vi "Sorted Particle Report.vi"(3 "Min Area Size %":dbl, 4 "Particle Count Limit":i32=2147483647, 5 "Pixel Measurements":T2[](array[typedef])=[35, 4, 5, 6, 7] items=["Center of Mass X", "Center of Mass Y", "First Pixel X", "First Pixel Y", "Bounding Rect Left", "Bounding Rect Top", "Bounding Rect Right", "Bounding Rect Bottom", "Max Feret Diameter Start X", "Max Feret Diameter Start Y", "Max Feret Diameter End X", "Max Feret Diameter End Y", "Max Horiz. Segment Length Left", "Max Horiz. Segment Length Right", "Max Horiz. Segment Length Row", "-", "Bounding Rect Width", "Bounding Rect Height", "Bounding Rect Diagonal", "Perimeter", "Convex Hull Perimeter", "Holes' Perimeter", "Max Feret Diameter", "Equivalent Ellipse Major Axis", "Equivalent Ellipse Minor Axis", "Equivalent Ellipse Minor Axis (Feret)", "Equivalent Rect Long Side", "Equivalent Rect Short Side", "Equivalent Rect Diagonal", "Equivalent Rect Short Side (Feret)", "Average Horiz. Segment Length", "Average Vert. Segment Length", "Hydraulic Radius", "Waddel Disk Diameter", "-", "Area", "Holes' Area", "Particle & Holes' Area", "Convex Hull Area", "Image Area", "-", "Number of Holes", "Number of Horiz. Segments", "Number of Vert. Segments", "-", "Orientation", "Max Feret Diameter Orientation", "-", "% Area/Image Area", "% Area/(Particle & Holes' Area)", "Ratio of Equivalent Ellipse Axes", "Ratio of Equivalent Rect Sides", "-", "Elongation Factor", "Compactness Factor", "Heywood Circularity Factor", "Type Factor", "-", "Sum X", "Sum Y", "Sum XX", "Sum XY", "Sum YY", "Sum XXX", "Sum XXY", "Sum XYY", "Sum YYY", "-", "Moment of Inertia XX", "Moment of Inertia XY", "Moment of Inertia YY", "Moment of Inertia XXX", "Moment of Inertia XXY", "Moment of Inertia XYY", "Moment of Inertia YYY", "Norm. Moment of Inertia XX", "Norm. Moment of Inertia XY", "Norm. Moment of Inertia YY", "Norm. Moment of Inertia XXX", "Norm. Moment of Inertia XXY", "Norm. Moment of Inertia XYY", "Norm. Moment of Inertia YYY", "Hu Moment 1", "Hu Moment 2", "Hu Moment 3", "Hu Moment 4", "Hu Moment 5", "Hu Moment 6", "Hu Moment 7"], 6 "Image in":T3) -> (0 "limits":T1, 1 "Sorted Data":dbl[][](array[numeric]), 2 "Particles":i32)   [LabVIEW 2019]
doc: "Returns the requested measurements of a binary image sorted by the first parameter (often size), and limiting the rows in the 2D array by count and by size. Pass infinity to count to avoid a limit. Pass zero to size to avoid a limit."
uses:
  <vilib>/vision/Image Controls.llb/IMAQ Image.ctl
  <vilib>/vision/NI_Vision_Development_Module.lvlib
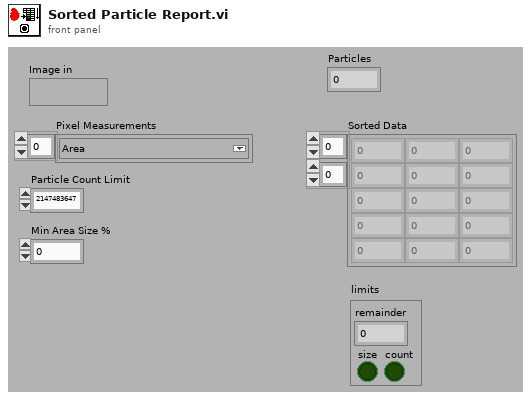
[diagram p1: front panel]
types:
  T1 = cluster{"remainder":i32, "size":bool, "count":bool}
  T2 = typedef "Particle Parameters" = i32
  T3 = typedef "IMAQ Image.ctl" = refnum<image>
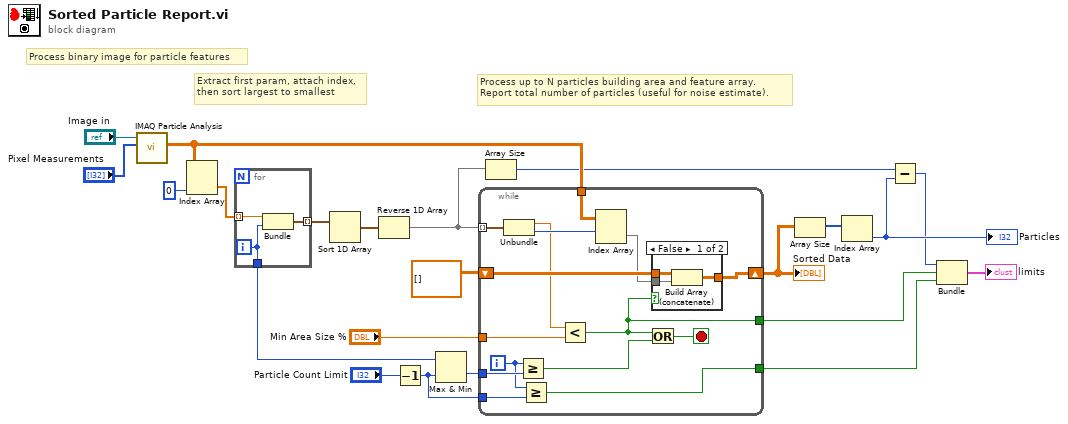
[diagram p0: block diagram]
diagram:
  # "Process up to N particles building area and feature array.\nReport total number of particles (useful for noise estimate)."
  # "Process binary image for particle features"
  # "Extract first param, attach index,\nthen sort largest to smallest"
  n1 = call "IMAQ Particle Analysis"("Pixel Measurements"="Pixel Measurements", "Image"="Image in") -> ("Particle Measurements (Pixels)"=w16:dbl[][])  [unwired: 3 in, 6 out]
  n2 = Index Array(array=w16, index (col)=0 ("disabled index (col)")) -> (element=w19:dbl[])  [unwired: 1 in]
  n3 = for {
    tunnel: w19 -> [w25] mode=indexing
    tunnel: [w24] -> w20 mode=indexing
    tunnel: [w23] -> w9
    i -> [w23]
    n4 = Bundle("Numeric"=w25, w23) -> (w24:cluster{"Numeric":dbl, i32})  [unwired: 1 out]
  }
  n5 = Sort 1D Array(array=w20) -> (sorted array=w21:cluster{"Numeric":dbl, i32}[])
  n6 = Reverse 1D Array(array=w21) -> (reversed array=w8:cluster{"Numeric":dbl, i32}[])
  n7 = Decrement(x="Particle Count Limit") -> (x-1=w1:i32)
  n8 = Max & Min(x=w9, y=w1) -> (min(x,y)=w10:i32)  [unwired: 1 out]
  n9 = while {
    tunnel: w16 -> [w39]
    tunnel: w8 -> [w38] mode=indexing
    shift-right: [w35] -> w12
    shift-left: dbl[][] [] -> [w37]
    tunnel: w10 -> [w34]
    tunnel: "Min Area Size %" -> [w32]
    tunnel: [w26] -> w3
    tunnel: [w29] -> w4
    tunnel: w1 -> [w28]
    i -> [w27]
    stop <- w31 stop-if-true
    n10 = Unbundle(w38) -> ("Numeric"=w33:dbl, w40:i32)
    n11 = Greater Or Equal?(x=w27, y=w34) -> (x >= y?=w30:bool)
    n12 = Greater Or Equal?(x=w27, y=w28) -> (x >= y?=w26:bool)
    n13 = Less?(x=w33, y=w32) -> (x < y?=w29:bool)
    n14 = Index Array(array=w39, index (row)=w40) -> (element=w36:dbl[])  [unwired: 1 in]
    n15 = Or(x=w29, y=w30) -> (x .or. y?=w31:bool)
    n16 = case shown="False" w29 {
      tunnel: w37 -> [w43 w44]
      tunnel: w36 -> [w42 _]
      tunnel: [w41 w44] -> w35
      frame False {
        n17 = Build Array (concatenate)(w43, w42) -> (w41:dbl[][])
      }
      frame True {
      }
    }
  }
  "Sorted Data" <- w12
  n18 = Array Size(array=w8) -> (size(s)=w6:i32)
  n19 = Array Size(array=w12) -> (size(s)=w11:i32[])
  n20 = Index Array(array=w11) -> (element=w7:i32)  [unwired: 1 in]
  "Particles" <- w7
  n21 = Subtract(x=w6, y=w7) -> (x-y=w5:i32)
  n22 = Bundle(w5, w4, w3) -> (→"limits":cluster{i32, bool, bool})  [unwired: 1 in]
